vi "AjustFrequency.vi"(11 "Frequency":dbl) -> (2 "N elements":i32, 3 "dt":i64)   [LabVIEW 2019]
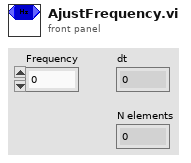
[diagram p1: front panel]
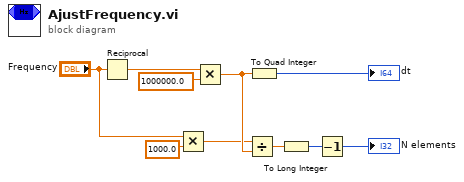
[diagram p0: block diagram]
diagram:
  n1 = Reciprocal(x="Frequency") -> (1/x=w8:dbl)
  n2 = Multiply(x="Frequency", y=1000.0) -> (x*y=w1:dbl)
  n3 = Multiply(x=w8, y=1000000.0) -> (x*y=w6:dbl)
  n4 = Divide(x=w1, y=w6) -> (x/y=w3:dbl)
  n5 = To Quad Integer(1:w6) -> (0:→"dt":i64)
  n6 = To Long Integer(number=w3) -> (32bit integer=w7:i32)
  n7 = Decrement(x=w7) -> (x-1=→"N elements":i32)
